vi "fgv_freq_real_imag.vi"(8 "Error in":errorcluster, 9 "mode":string(combo)="Get", 10 "data_array_set":dbl[][](array[numeric]), 11 "freq_array_set":dbl[](array[numeric])) -> (0 "error out":errorcluster, 1 "plot_data":T1(array[cluster]), 2 "data_array_get":dbl[][](array[numeric]), 3 "freq_array_get":dbl[](array[numeric]))   [LabVIEW 2025]
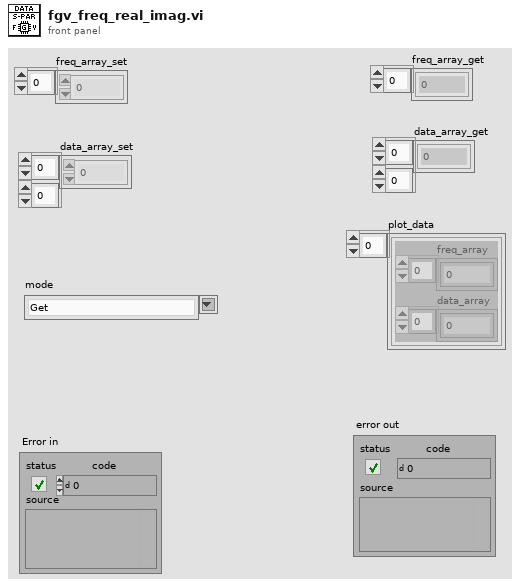
[diagram p1: front panel]
types:
  T1 = cluster{"freq_array":dbl[], "data_array":dbl[]}[]
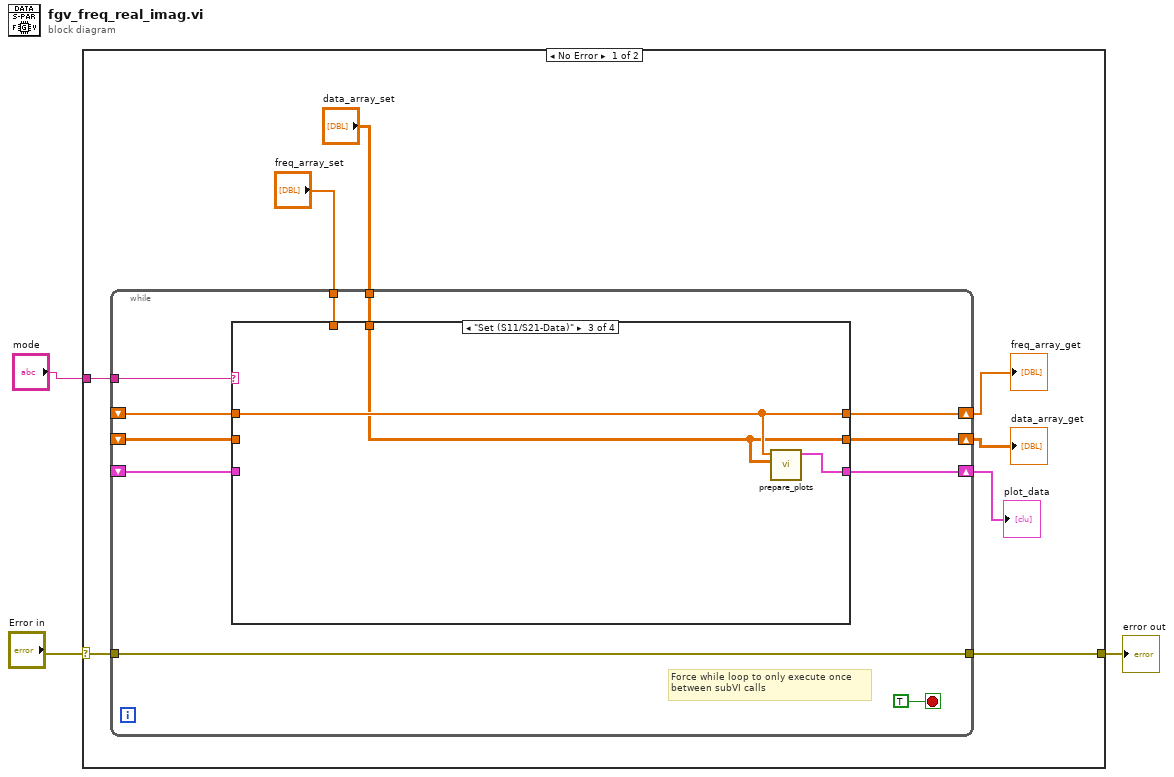
[diagram p0: block diagram]
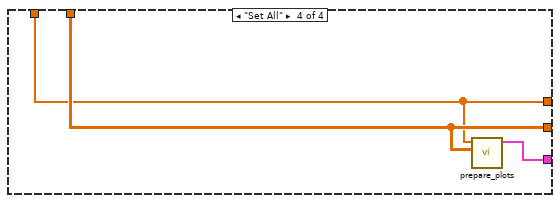
[diagram p4: hidden frame]
diagram:
  n1 = case shown="No Error" "Error in" {
    selector: "Error in" -> [w11 w35]
    tunnel: [w10 w35] -> w2
    tunnel: "mode" -> [w9 _]
    frame No Error {
      n2 = while {
        shift-right: [w20] -> w6
        shift-left: _ -> [w21]
        shift-right: [w19] -> w8
        shift-left: _ -> [w18]
        tunnel: w11 -> [w17]
        tunnel: [w17] -> w10
        tunnel: w9 -> [w16]
        shift-right: [w15] -> w7
        shift-left: _ -> [w14]
        tunnel: "freq_array_set" -> [w13]
        tunnel: "data_array_set" -> [w12]
        stop <- TRUE stop-if-true
        # "Force while loop to only execute once\nbetween subVI calls"
        n3 = case shown="\"Set (S11/S21-Data)\"" w16 {
          tunnel: w21 -> [w24 _ w30 _]
          tunnel: [w24 w28 w30 w32] -> w20
          tunnel: [w25 w27 w29 w33] -> w19
          tunnel: w18 -> [w25 w27 _ _]
          tunnel: [w23 w26 w31 w34] -> w15
          tunnel: w14 -> [w23 w26 _ _]
          tunnel: w13 -> [_ w28 _ w32]
          tunnel: w12 -> [_ _ w29 w33]
          frame "Get", Default {
          }
          frame "Set (Frequencies)" {
          }
          frame "Set (S11/S21-Data)" {
            n4 = call "prepare_plots.vi"("data_array"=w29, "freq_array"=w30) -> ("plot_data"=w31:cluster{"freq_array":dbl[], "X2":dbl[]}[])  [unwired: 9 in]
          }
          frame "Set All" {
            n5 = call "prepare_plots.vi"("data_array"=w33, "freq_array"=w32) -> ("plot_data"=w34:cluster{"freq_array":dbl[], "X2":dbl[]}[])  [unwired: 9 in]
          }
        }
      }
      "data_array_get" <- w8
      "freq_array_get" <- w6
      "plot_data" <- w7
    }
    frame Error {
      # "Case structure checks for errors - if there's an errorr, do nothing except pass the error back out"
    }
  }
  "error out" <- w2
